vi "Get Specific Filter Configuration String.vi"(11 "Base Filter in":refnum<class "Base Filter.lvclass">) -> (2 "Filter String":string)   [LabVIEW 2016, in "Assert API Components.lvlib" / "Base Filter.lvclass"]
uses:
  Base Filter.lvclass
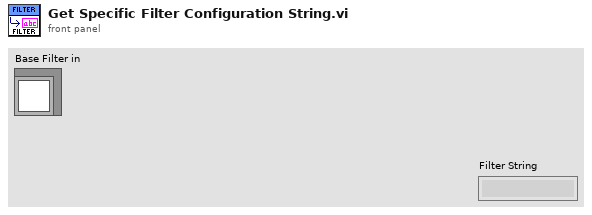
[diagram p1: front panel]
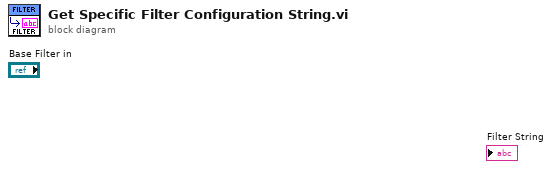
[diagram p0: block diagram]
diagram:
